vi "3.1--Genereate Function.vi"(1 "Left Data":T1, 2 "Right Data":T1) -> (0 "Function":dbl[](array[numeric]))   [LabVIEW 2010]
panel:
  out "size(s)":i32
  out "XY Graph":cluster{dbl[], dbl[]}(graph)
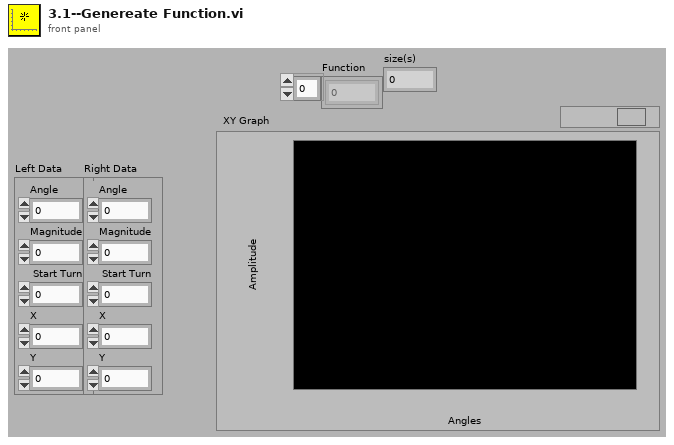
[diagram p1: front panel]
types:
  T1 = cluster{"Angle":dbl, "Magnitude":dbl, " Start Turn":dbl, "X":dbl, "Y":dbl}
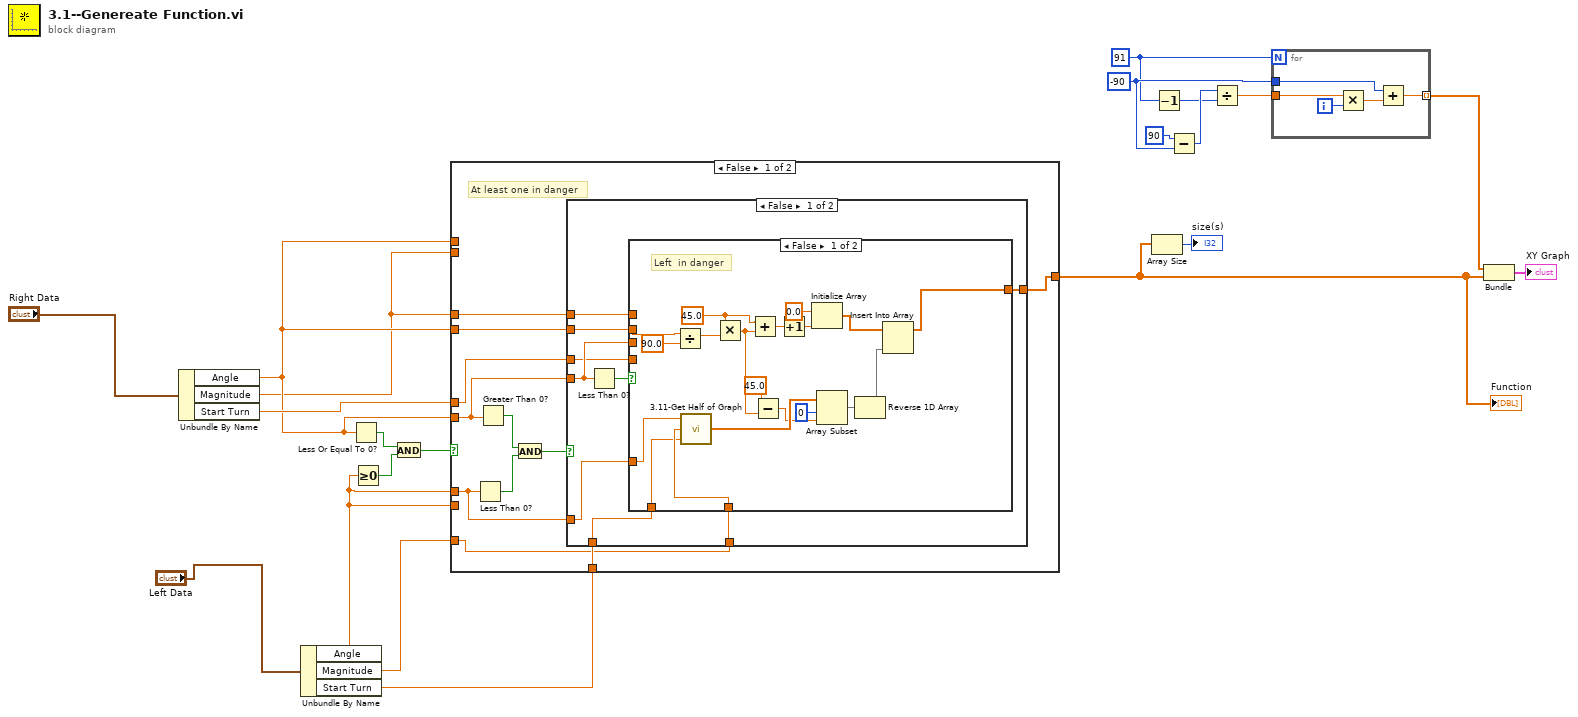
[diagram p0: block diagram]
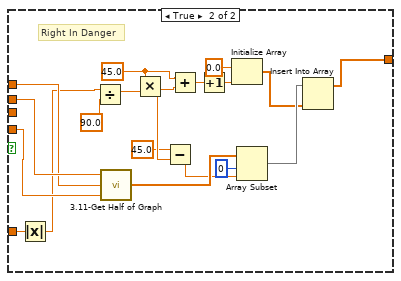
[diagram p2: hidden frame]
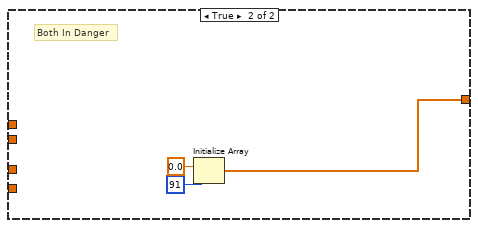
[diagram p3: hidden frame]
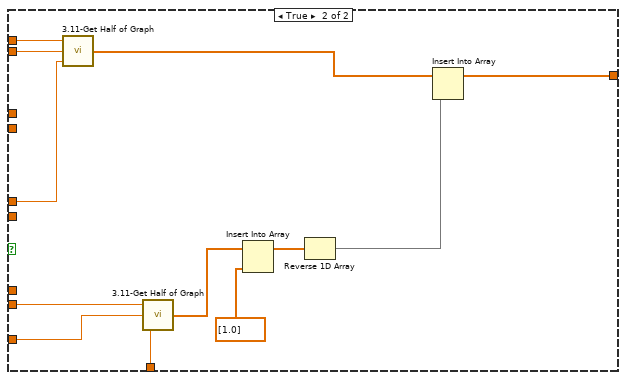
[diagram p4: hidden frame]
diagram:
  w17 = -90
  w15 = 91 ("samples")
  n1 = Unbundle By Name("Right Data") -> ("Angle"=w6:dbl, "Magnitude"=w5:dbl, "Start Turn"=w11:dbl)
  n2 = Unbundle By Name("Left Data") -> ("Angle"=w7:dbl, "Magnitude"=w21:dbl, "Start Turn"=w12:dbl)
  n3 = Less Or Equal To 0?(x=w6) -> (x <= 0?=w10:bool)
  n4 = Greater Or Equal To 0?(x=w7) -> (x >= 0?=w9:bool)
  n5 = And(x=w10, y=w9) -> (x .and. y?=w8:bool)
  n6 = case shown="False" w8 {
    tunnel: w21 -> [w23 w94]
    tunnel: [w29 w93] -> w4
    tunnel: w7 -> [_ w92]
    tunnel: w12 -> [w25 w91]
    tunnel: w6 -> [_ w88]
    tunnel: w5 -> [_ w87]
    tunnel: w11 -> [w22 w86]
    tunnel: w7 -> [w27 _]
    tunnel: w6 -> [w28 _]
    tunnel: w6 -> [w26 _]
    tunnel: w5 -> [w24 _]
    frame False {
      # "At least one in danger"
      n7 = Less Than 0?(x=w27) -> (x < 0?=w32:bool)
      n8 = Greater Than 0?(x=w28) -> (x > 0?=w31:bool)
      n9 = And(x=w31, y=w32) -> (x .and. y?=w30:bool)
      n10 = case shown="False" w30 {
        tunnel: [w33 w80] -> w29
        tunnel: w28 -> [w40 _]
        tunnel: w27 -> [w37 _]
        tunnel: w26 -> [w39 _]
        tunnel: w25 -> [w38 _]
        tunnel: w24 -> [w36 _]
        tunnel: w23 -> [w35 _]
        tunnel: w22 -> [w34 _]
        frame False {
          n11 = Less Than 0?(x=w40) -> (x < 0?=w41:bool)
          n12 = case shown="False" w41 {
            tunnel: w40 -> [_ _]
            tunnel: w39 -> [w60 w71]
            tunnel: w38 -> [w52 _]
            tunnel: w37 -> [w54 w72]
            tunnel: w36 -> [_ w70]
            tunnel: w35 -> [w53 _]
            tunnel: w34 -> [_ w69]
            tunnel: [w48 w66] -> w33
            frame False {
              w57 = 45.0 ("x")
              # "Left  in danger"
              n13 = Divide(x=w60, y=90.0) -> (x/y=w58:dbl)
              n14 = call "3.11-Get Half of Graph.vi"("Start Turn"=w52, "Magnitude"=w53, "Angle"=w54) -> ("Array"=w50:dbl[])
              n15 = Multiply(x=w57, y=w58) -> (x*y=w47:dbl)
              n16 = Add(x=w57, y=w47) -> (x+y=w49:dbl)
              n17 = Subtract(x=45.0, y=w47) -> (x-y=w44:dbl)
              n18 = Increment(x=w49) -> (x+1=w55:dbl)
              n19 = Initialize Array(0.0 ("element"), w55) -> (w51:dbl[])
              n20 = Array Subset(array=w50, index=0, length=w44) -> (w45:dbl[])
              n21 = Reverse 1D Array(array=w45) -> (reversed array=w42:dbl[])
              n22 = Insert Into Array(array=w51, new element=w42) -> (w48:dbl[])  [unwired: 1 in]
            }
            frame True {
              w77 = 45.0 ("x")
              # "Right In Danger"
              n23 = Absolute Value(x=w72) -> (abs(x)=w65:dbl)
              n24 = Divide(x=w65, y=90.0) -> (x/y=w78:dbl)
              n25 = call "3.11-Get Half of Graph.vi"("Start Turn"=w69, "Magnitude"=w70, "Angle"=w71) -> ("Array"=w74:dbl[])
              n26 = Multiply(x=w77, y=w78) -> (x*y=w62:dbl)
              n27 = Subtract(x=45.0, y=w62) -> (x-y=w63:dbl)
              n28 = Add(x=w77, y=w62) -> (x+y=w73:dbl)
              n29 = Increment(x=w73) -> (x+1=w75:dbl)
              n30 = Initialize Array(0.0 ("element"), w75) -> (w67:dbl[])
              n31 = Array Subset(array=w74, index=0, length=w63) -> (w68:dbl[])
              n32 = Insert Into Array(array=w68, new element=w67) -> (w66:dbl[])  [unwired: 1 in]
            }
          }
        }
        frame True {
          # "Both In Danger"
          n33 = Initialize Array(0.0 ("element"), 91 ("dimension size")) -> (w80:dbl[])
        }
      }
    }
    frame True {
      n34 = call "3.11-Get Half of Graph.vi"("Start Turn"=w86, "Magnitude"=w87, "Angle"=w88) -> ("Array"=w83:dbl[])
      n35 = call "3.11-Get Half of Graph.vi"("Start Turn"=w91, "Magnitude"=w94, "Angle"=w92) -> ("Array"=w90:dbl[])
      n36 = Insert Into Array(array=w90, new element=dbl[] [1.0] ("array")) -> (w85:dbl[])  [unwired: 1 in]
      n37 = Reverse 1D Array(array=w85) -> (reversed array=w84:dbl[])
      n38 = Insert Into Array(array=w83, new element=w84) -> (w93:dbl[])  [unwired: 1 in]
    }
  }
  "Function" <- w4
  n39 = Array Size(array=w4) -> (size(s)=→"size(s)":i32)
  n40 = Decrement(x=w15) -> (x-1=w16:i32)
  n41 = Subtract(x=90, y=w17) -> (x-y=w20:i32)
  n42 = Divide(x=w20, y=w16) -> (x/y=w19:dbl)
  n43 = for {
    N: w15 -> [_]
    tunnel: w19 -> [w98]
    tunnel: w17 -> [w96]
    tunnel: [w95] -> w14 mode=indexing
    i -> [w99]
    n44 = Multiply(x=w98, y=w99) -> (x*y=w97:dbl)
    n45 = Add(x=w96, y=w97) -> (x+y=w95:dbl)
  }
  n46 = Bundle(w14, "Array"=w4) -> (→"XY Graph":cluster{dbl[], "Array":dbl[]})  [unwired: 1 in]
